vi "Update.vi"(8 "error in (no error)":errorcluster, 10 "Message in":refnum<class "UpdateMessage.lvclass">=refnum, 11 "Cobolt in":refnum<class "Cobolt.lvclass">) -> (0 "error out":errorcluster, 3 "Cobolt out":refnum<class "Cobolt.lvclass">)   [LabVIEW 2012, in "Cobolt.lvclass"]
doc: "The update method processes the command 'update'. \n\nThe command 'update' is used for receiving new values to be set to the private data of the class. This could be seen as a public set method for setting new parameters to the private class data."
uses:
  Cobolt.lvclass
  <vilib>/Distrio/Murmex/UpdateMessage/UpdateMessage.lvclass
  <vilib>/Distrio/Murmex/Murmex/Murmex.lvclass
  Murmex/LabVIEW/Murmex/UpdateMessage/UpdateMessage.lvclass
panel:
  # "This method is called when the UPDATE\ntrigger is sent. \n\nOverride this method when your component needs to\nrespond to this trigger. \n\nCall parent for proper implementation"
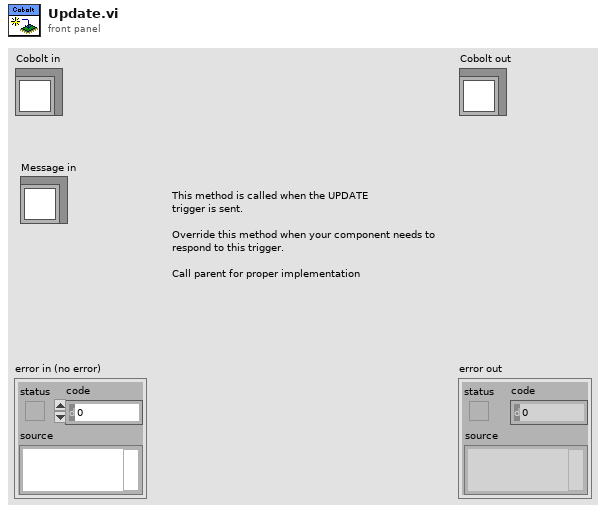
[diagram p1: front panel]
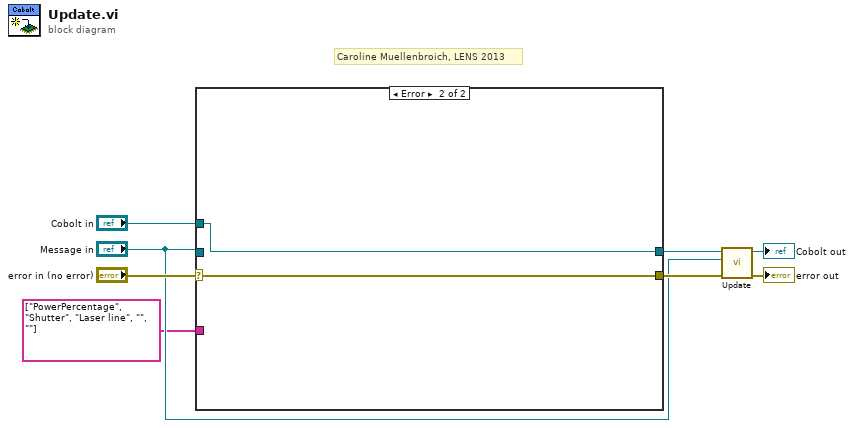
[diagram p0: block diagram]
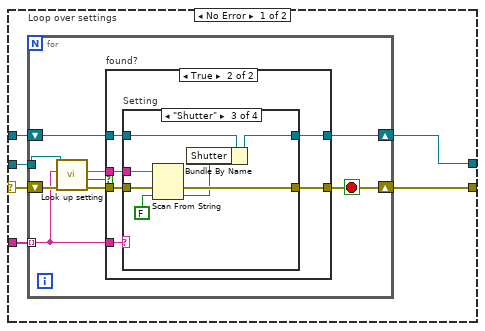
[diagram p2: hidden frame]
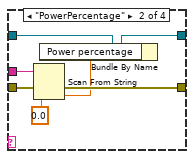
[diagram p5: hidden frame]
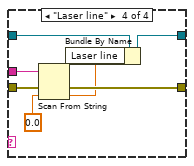
[diagram p6: hidden frame]
diagram:
  # "Caroline Muellenbroich, LENS 2013"
  n1 = case shown="Error" "error in (no error)" {
    selector: "error in (no error)" -> [w14 w56]
    tunnel: "Message in" -> [w13 _]
    tunnel: "Cobolt in" -> [w12 w55]
    tunnel: [w10 w56] -> w6
    tunnel: [w11 w55] -> w2
    tunnel: string[] ["PowerPercentage", "Shutter", "Laser line", "", ""] ("key chains") -> [w9 _]
    frame No Error {
      n2 = for "Loop over settings" {
        shift-right: [w16] -> w10
        shift-left: w14 -> [w23]
        tunnel: w13 -> [w22]
        shift-right: [w17] -> w11
        shift-left: w12 -> [w20]
        tunnel: w9 -> [w15] mode=indexing
        stop <- w16 stop-if-true
        n3 = call <vilib>:"Look up setting.vi"("error in (no error)"=w23, "tag name"=w15, "UpdateMessage in"=w22) -> ("error out"=w18:errorcluster, "found?"=w21:bool, "value"=w19:string)  [unwired: 5 in, 1 out]
        n4 = case "found?" shown="True" w21 {
          tunnel: w20 -> [w25 w30]
          tunnel: w19 -> [_ w31]
          tunnel: w18 -> [w24 w29]
          tunnel: [w25 w28] -> w17
          tunnel: [w24 w27] -> w16
          tunnel: w15 -> [_ w26]
          frame False {
          }
          frame True {
            n5 = case "Setting" shown="\"Shutter\"" w26 {
              tunnel: w31 -> [_ w35 w45 w52]
              tunnel: w30 -> [w33 w39 w44 w51]
              tunnel: w29 -> [w32 w40 w47 w54]
              tunnel: [w33 w38 w43 w50] -> w28
              tunnel: [w32 w36 w46 w53] -> w27
              frame Default {
              }
              frame "PowerPercentage" {
                n6 = Scan From String(input string=w35, error in=w40, default 1=0.0 ("Settings_cluster.Power")) -> (error out=w36:errorcluster, output 1=w34:dbl)  [unwired: 2 in, 2 out]
                n7 = Bundle By Name(cluster=w39, "Power percentage"=w34) -> (w38:refnum<class "Cobolt.lvclass">)
              }
              frame "Shutter" {
                n8 = Scan From String(input string=w45, error in=w47, default 1=FALSE ("settings.Shutter")) -> (error out=w46:errorcluster, output 1=w41:bool)  [unwired: 2 in, 2 out]
                n9 = Bundle By Name(cluster=w44, "Shutter"=w41) -> (w43:refnum<class "Cobolt.lvclass">)
              }
              frame "Laser line" {
                n10 = Scan From String(input string=w52, error in=w54, default 1=0.0 ("settings.Laser line")) -> (error out=w53:errorcluster, output 1=w49:dbl)  [unwired: 2 in, 2 out]
                n11 = Bundle By Name(cluster=w51, "Laser line"=w49) -> (w50:refnum<class "Cobolt.lvclass">)
              }
            }
          }
        }
      }
    }
    frame Error {
    }
  }
  n12 = call-parent "Update.vi"("error in (no error)"=w6, "Message in"="Message in", "Murmex in"=w2) -> ("error out"=→"error out":errorcluster, "Murmex out"=→"Cobolt out":refnum<class "Cobolt.lvclass">)  [unwired: 7 in]
